vi "Start Measurement.vi"(7 "Start new file":bool=TRUE, 8 "error in (no error)":errorcluster, 10 "Save data settings":T1={"Save data"=TRUE, "Data Root Path"=path "", "File Prefix"="", "File Format"=enum."ASCII", "Save column names"=TRUE, "File Comments"="<Description of the current file>", "User/Prj"="<User Name/Project Description>"}, 11 "Devices":refnum<class "Device.lvclass">[](array[class])) -> (0 "error out":errorcluster, 1 "Columns":string, 2 "Save data settings out":T1={"Save data"=TRUE, "Data Root Path"=path "", "File Prefix"="", "File Format"=enum."ASCII", "Save column names"=TRUE, "File Comments"="<Description of the current file>", "User/Prj"="<User Name/Project Description>"}, 3 "Devices out":refnum<class "Device.lvclass">[](array[class]), 4 "Settings":string, 5 "Data titles":string[](array[string]))   [LabVIEW 2015]
uses:
  Device/Device.lvclass
  File/Controls/File formats.ctl
  File/Controls/Save data settings.ctl
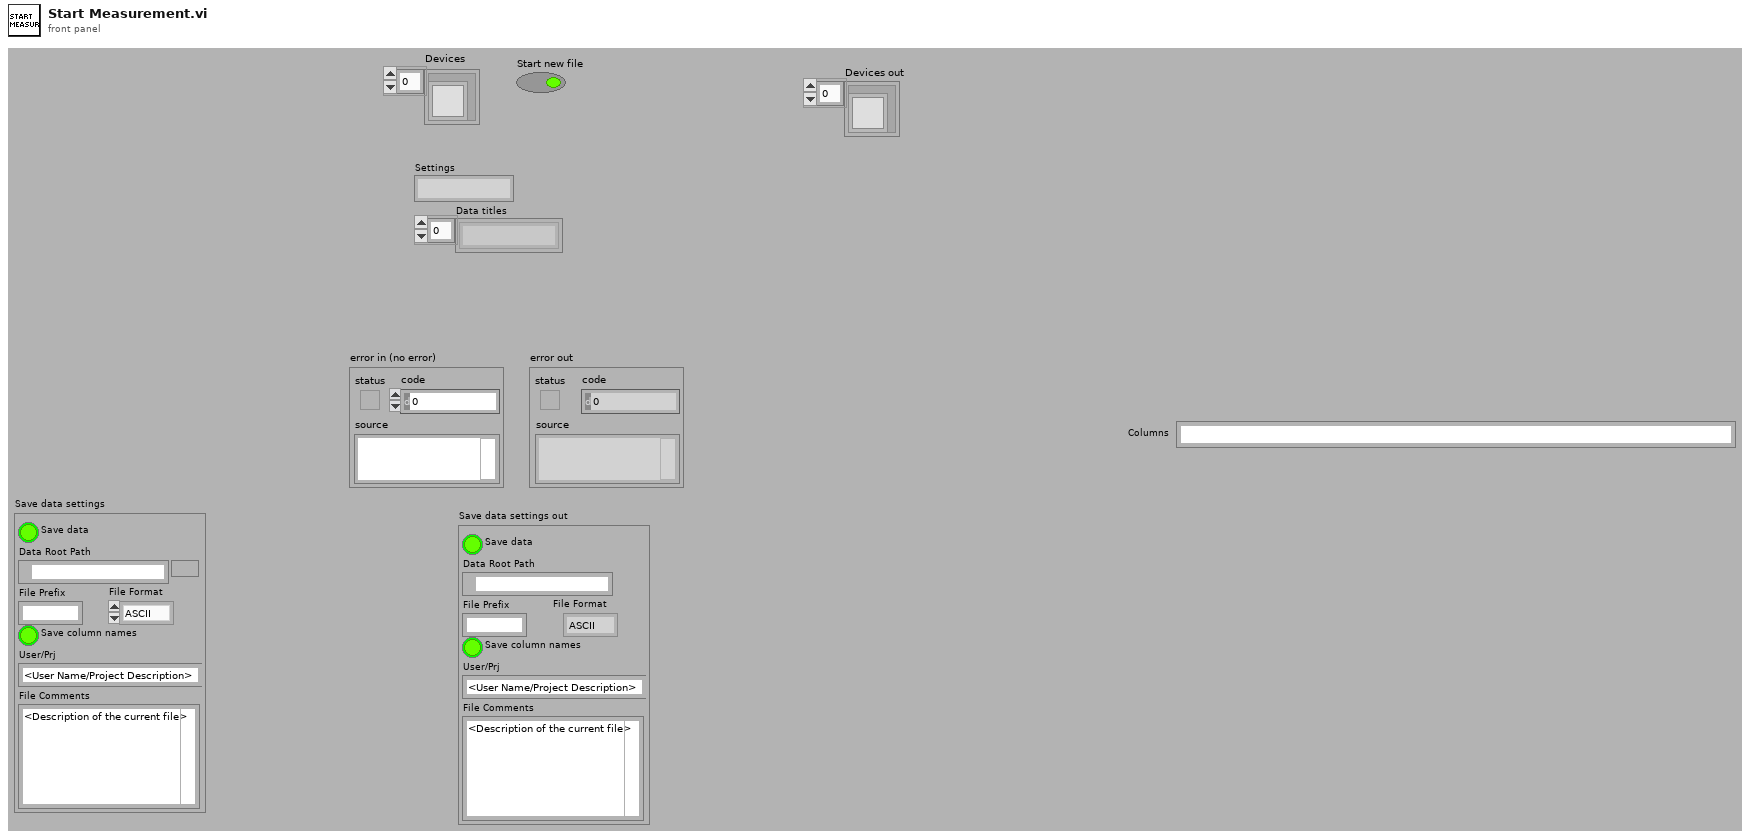
[diagram p1: front panel]
types:
  T1 = typedef "Save data settings.ctl" = cluster{"Save data":bool, "Data Root Path":path, "File Prefix":string, "File Format":T2, "Save column names":bool, "File Comments":string, "User/Prj":string}
  T2 = typedef "File formats.ctl" = enum16{"TDMS", "ASCII", "BINARY"}
  T3 = enum16{"Set", "Get", "Set Instruments", "Set active state"}
  T4 = cluster{"Measurements active":bool, "Instruments":refnum<class "Device.lvclass">[], "Save data settings":T1, "Start time":u32}
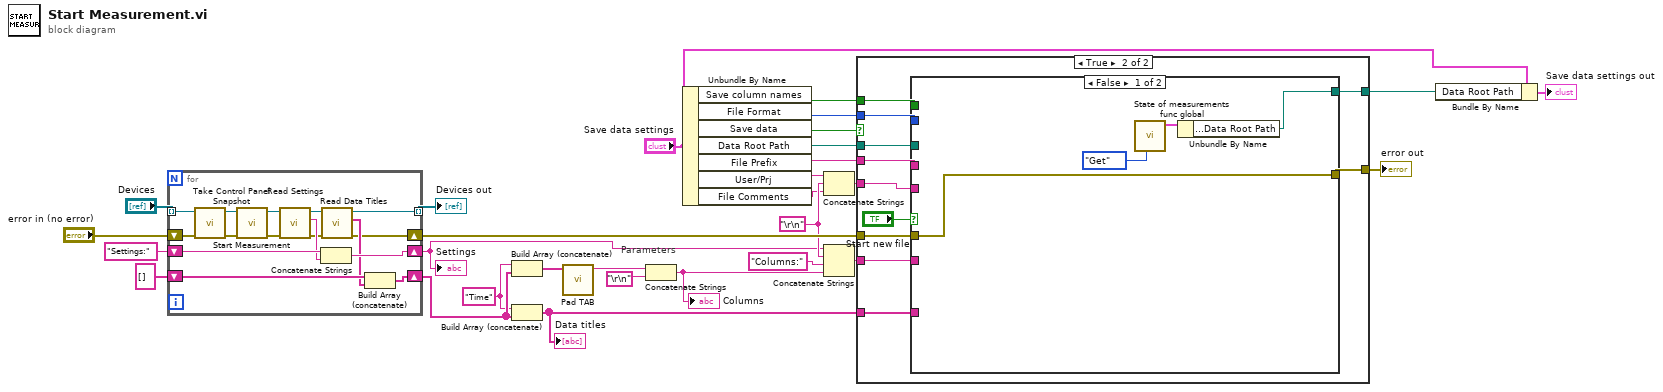
[diagram p0: block diagram]
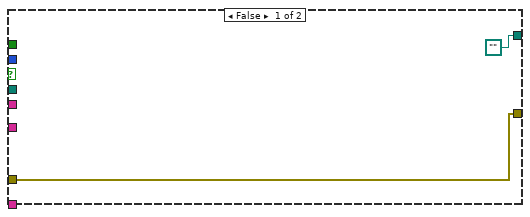
[diagram p2: hidden frame]
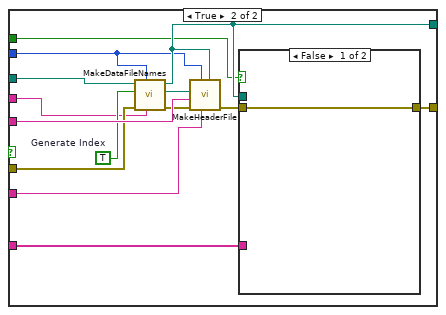
[diagram p3: hidden frame]
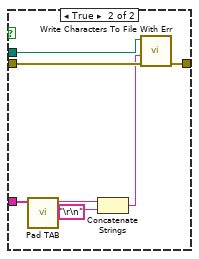
[diagram p4: hidden frame]
diagram:
  w20 = "\r\n"
  w4 = "Time"
  # "Parameters"
  n1 = for {
    shift-right: [w43] -> w17
    shift-left: "Settings:" -> [w42]
    shift-right: [w38] -> w25
    shift-left: "error in (no error)" -> [w39]
    shift-right: [w45] -> w16
    shift-left: string[] [] ("Data titles") -> [w44]
    tunnel: "Devices" -> [w36] mode=indexing
    tunnel: [w37] -> w27 mode=indexing
    n2 = call-dynamic "Take Control Panel Snapshot.vi"("error in (no error)"=w39, "Device in"=w36) -> ("error out"=w32:errorcluster, "Device out"=w31:refnum<class "Device.lvclass">)  [unwired: 7 in, 1 out]
    n3 = call-dynamic "Start Measurement.vi"("error in (no error)"=w32, "Device in"=w31) -> ("error out"=w33:errorcluster, "Device out"=w30:refnum<class "Device.lvclass">)  [unwired: 8 in]
    n4 = call-dynamic "Read Settings.vi"("error in (no error)"=w33, "Device in"=w30) -> ("error out"=w35:errorcluster, "Settings"=w40:string, "Device out"=w34:refnum<class "Device.lvclass">)  [unwired: 1 in, 6 out]
    n5 = Concatenate Strings(w42, w40) -> (w43:string)
    n6 = call-dynamic "Read Data Titles.vi"("error in (no error)"=w35, "Device in"=w34) -> ("error out"=w38:errorcluster, "Data titles"=w41:string[], "Device out"=w37:refnum<class "Device.lvclass">)  [unwired: 7 out]
    n7 = Build Array (concatenate)(w44, w41) -> (w45:string[])
  }
  "Settings" <- w17
  "Devices out" <- w27
  n8 = Build Array (concatenate)(w4, w16) -> (w22:string[])
  n9 = Build Array (concatenate)(w4, w16) -> (w5:string[])
  "Data titles" <- w5
  n10 = call "Pad TAB.vi"("Input String Array"=w22) -> ("Output String"=w3:string)  [unwired: 3 in, 7 out]
  n11 = Concatenate Strings(w3, "\r\n") -> (w2:string)
  "Columns" <- w2
  n12 = Unbundle By Name("Save data settings") -> ("Save column names"=w9:bool, "File Format"=w13:T2, "Save data"=w15:bool, "Data Root Path"=w14:path, "File Prefix"=w12:string, "User/Prj"=w11:string, "File Comments"=w10:string)
  n13 = Concatenate Strings(w11, w20, w10) -> (w19:string)
  n14 = Concatenate Strings(w17, w20, "Columns:", w2) -> (w18:string)
  n15 = case shown="True" w15 {
    tunnel: w25 -> [w47 w54]
    tunnel: w18 -> [_ w58]
    tunnel: w19 -> [_ w57]
    tunnel: [w47 w55] -> w24
    tunnel: w5 -> [_ w56]
    tunnel: [path "" w53] -> w6
    tunnel: w14 -> [_ w52]
    tunnel: w13 -> [_ w51]
    tunnel: w12 -> [_ w50]
    tunnel: w9 -> [_ w49]
    frame False {
    }
    frame True {
      n16 = case shown="False" "Start new file" {
        tunnel: w58 -> [_ w76]
        tunnel: w57 -> [_ w75]
        tunnel: w56 -> [_ w74]
        tunnel: [w62 w72] -> w55
        tunnel: w54 -> [w62 w70]
        tunnel: [w59 w68] -> w53
        tunnel: w52 -> [_ w66]
        tunnel: w51 -> [_ w65]
        tunnel: w50 -> [_ w64]
        tunnel: w49 -> [_ w63]
        frame False {
          n17 = call "State of measurements func global.vi"("Operation"=T3."Get") -> ("Measurement settings out"=w60:T4)  [unwired: 10 in]
          n18 = Unbundle By Name(w60) -> ("Save data settings.Data Root Path"=w59:path)
        }
        frame True {
          w67 = TRUE  # Generate Index
          n19 = call "MakeDataFileNames.vi"("File Prefix"=w64, "File format"=w65, "error in (no error)"=w70, "Generate Index"=w67, "Root Data Folder"=w66) -> ("error out"=w69:errorcluster, "Settings File Path"=w71:path, "Data File  Path"=w68:path)  [unwired: 4 in]
          n20 = call "MakeHeaderFile.vi"("Data File Name 1"=w68, "Parameters"=w76, "File Format"=w65, "error in (no error)"=w69, "File Description"=w75, "File Name"=w71) -> ("error out"=w73:errorcluster)  [unwired: 2 in, 3 out]
          n21 = case shown="False" w63 {
            tunnel: w74 -> [_ w84]
            tunnel: w73 -> [w77 w83]
            tunnel: [w77 w82] -> w72
            tunnel: w68 -> [_ w78]
            frame False {
            }
            frame True {
              n22 = call "Pad TAB.vi"("Input String Array"=w84) -> ("Output String"=w81:string)  [unwired: 1 in, 9 out]
              n23 = Concatenate Strings(w81, "\r\n") -> (w80:string)
              n24 = call "Write Characters To File With Err.vi"("error in (no error)"=w83, "character string"=w80, "file path (dialog if empty)"=w78) -> ("error out"=w82:errorcluster)  [unwired: 2 in, 6 out]
            }
          }
        }
      }
    }
  }
  "error out" <- w24
  n25 = Bundle By Name(cluster="Save data settings", "Data Root Path"=w6) -> (→"Save data settings out":T1)
